vi "_Export Table To Text File.vi"(0 "delimiter (\\t)":string="\t", 1 "transpose? (no:F)":bool, 4 "format (%s)":string="%s", 5 "append to file? (new file:F)":bool, 6 "1D data":string[](array[string]), 7 "2D data":string[][](array[string]), 8 "file path (dialog if empty)":path) -> (3 "new file path (Not A Path if cancelled)":path)   [LabVIEW 2012]
doc: "Converts a 2D or 1D array of strings, signed integers, or double-precision numbers to a text string and writes the string to a new byte stream file or appends the string to an existing file. \n\nWire data to the <B>2D data</B> input or <B>1D data</B> input to determine the polymorphic instance to use or manually select the instance."
panel:
  in  "prompt":string="Choose file to write."
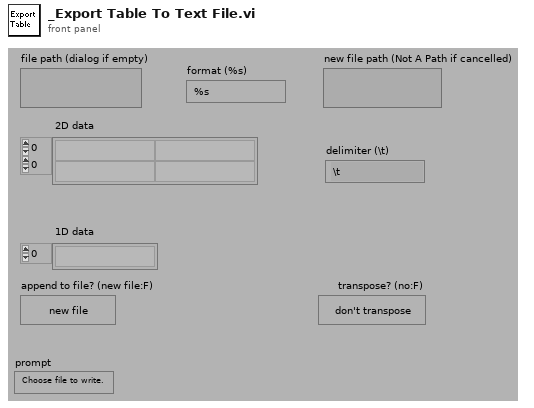
[diagram p1: front panel]
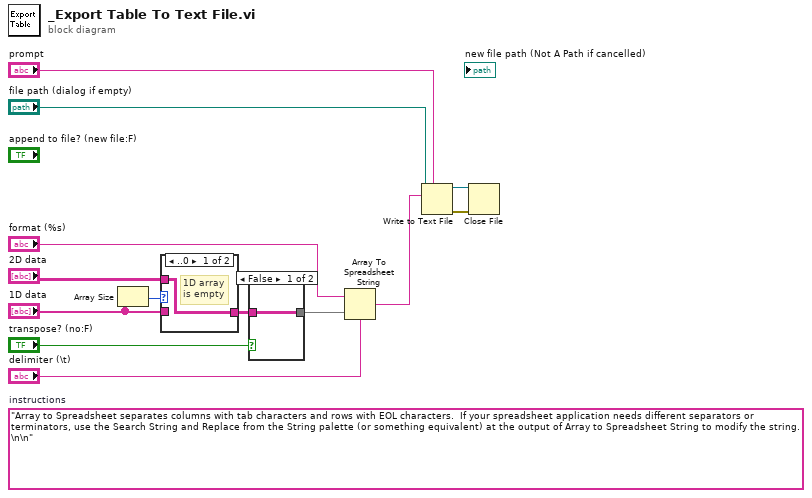
[diagram p0: block diagram]
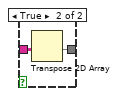
[diagram p2: hidden frame]
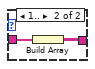
[diagram p3: hidden frame]
diagram:
  (unwired) "Array to Spreadsheet separates columns with tab characters and rows with EOL characters.  If your spreadsheet application needs different separators or terminators, use the Search String and Replace from the String palette (or something equivalent) at the output of Array to Spreadsheet String to modify the string.\n\n"  # instructions
  n1 = Array Size(array="1D data") -> (size(s)=w13:i32)
  n2 = case shown="..0" w13 {
    tunnel: "1D data" -> [_ w16]
    tunnel: [w14 w15] -> w9
    tunnel: "2D data" -> [w14 _]
    frame ..0 {
      # "1D array is empty"
    }
    frame 1.. {
      n3 = Build Array(w16) -> (w15:string[][])
    }
  }
  n4 = case shown="False" "transpose? (no:F)" {
    tunnel: [w17 w19] -> w7
    tunnel: w9 -> [w17 w18]
    frame False {
    }
    frame True {
      n5 = Transpose 2D Array(2D array=w18) -> (transposed array=w19:string[][])
    }
  }
  n6 = Array To Spreadsheet String(delimiter (Tab)="delimiter (\\t)", array=w7, 3:"format (%s)") -> (spreadsheet string=w4:string)
  n7 = Write to Text File(prompt (Choose or enter file path)="prompt", file (use dialog)="file path (dialog if empty)", text=w4) -> (refnum out=w2:refnum<file>, error out=w3:errorcluster)  [unwired: 1 in, 1 out]
  n8 = Close File(refnum=w2, error in=w3) -> ()  [unwired: 2 out]
